vi "Get Background.vi"(10 "X":dbl[](array[numeric]), 11 "Fit parameters":T1={"Peaks"=[{"Amplitude"=4000.0, "Center"=694.3, "Width"=0.4}, {"Amplitude"=2000.0, "Center"=692.8, "Width"=0.4}], "Slope"=nan, "Intercept"=0.0, "Function"=enum."Gauss"}) -> (2 "Y":dbl[](array[numeric]))   [LabVIEW 2016]
uses:
  Multi-peak Parameters.ctl
  Peak Parameters.ctl
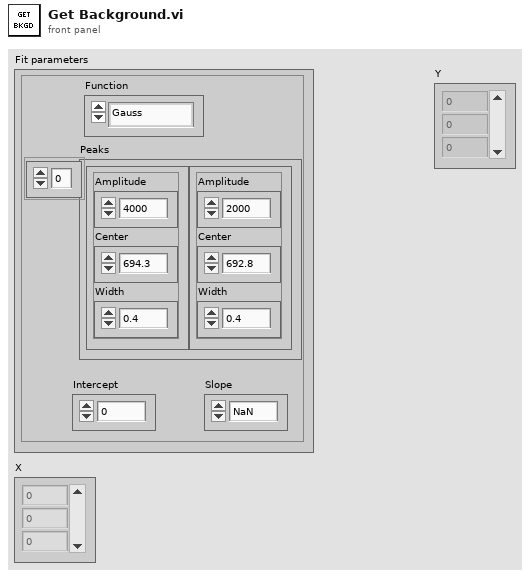
[diagram p1: front panel]
types:
  T1 = typedef "Multi-peak Parameters.ctl" = cluster{"Peaks":T2[], "Slope":dbl, "Intercept":dbl, "Function":enum16{"Gauss", "Lorentz"}}
  T2 = typedef "Peak Parameters.ctl" = cluster{"Amplitude":dbl, "Center":dbl, "Width":dbl}
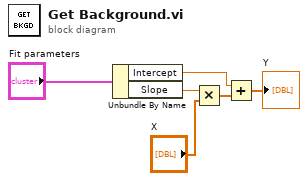
[diagram p0: block diagram]
diagram:
  n1 = Unbundle By Name("Fit parameters") -> ("Intercept"=w2:dbl, "Slope"=w4:dbl)
  n2 = Multiply(x=w4, y="X") -> (x*y=w3:dbl[])
  n3 = Add(x=w2, y=w3) -> (x+y=→"Y":dbl[])
